vi "Write Page Button List Properties.vi"(8 "Error In":errorcluster, 10 "Button List Properties":T1[](array[typedef]), 11 "Custom Device Page .NET Ref In":refnum<k24>) -> (0 "Error Out":errorcluster, 3 "Custom Device Page .NET Ref Out":refnum<k24>)   [LabVIEW 2015, in "VeriStand Custom Device XML Parser.lvlib"]
doc: "Sets the properties for each button and sets the array of button properties to the page"
uses:
  VeriStand Custom Device XML Parser.lvlib
  NationalInstruments.VeriStand.XMLReader
  XML Controls/ButtonLists Properties.ctl
  XML Controls/Path Cluster.ctl
  XML Controls/Button Type.ctl
  XML Controls/Dependency Properties.ctl
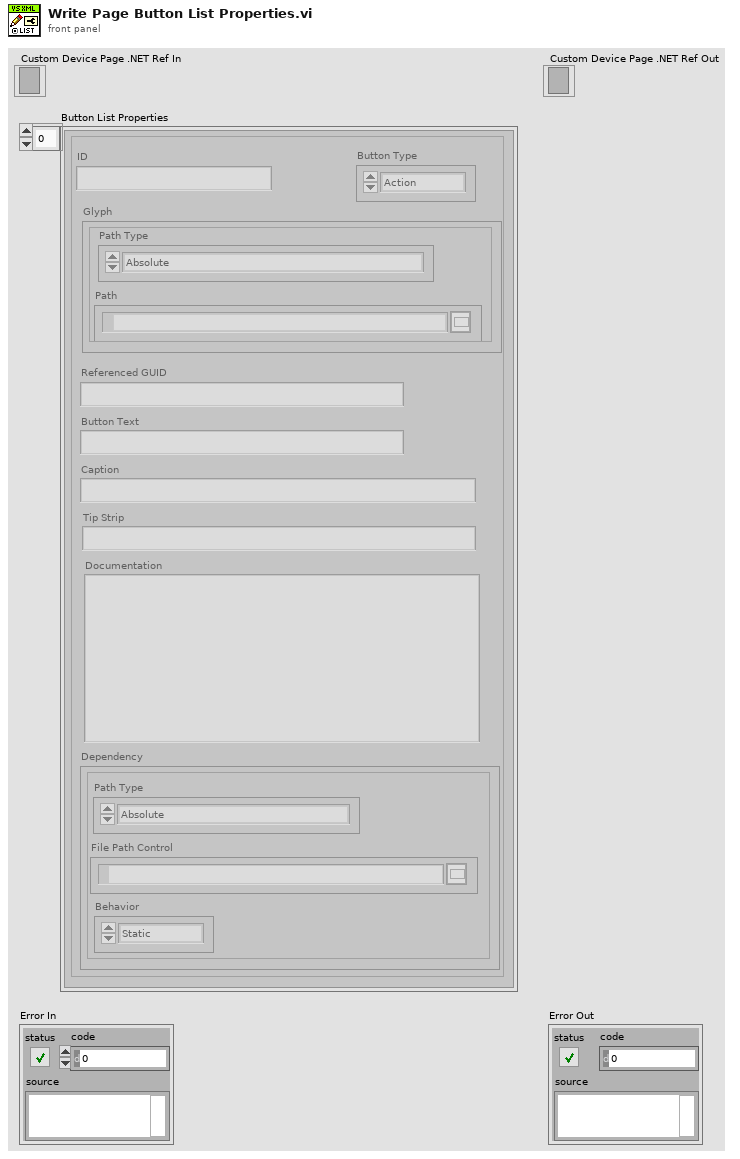
[diagram p1: front panel]
types:
  T1 = typedef "VeriStand Custom Device XML Parser.lvlib/ButtonLists Properties.ctl" = cluster{"ID":string, "Glyph":T2, "Button Type":T3, "Referenced GUID":string, "Button Text":string, "Caption":string, "Tip Strip":string, "Documentation":string, "Dependency":T4}
  T2 = typedef "VeriStand Custom Device XML Parser.lvlib/Path Cluster.ctl" = cluster{"Path":path, "Path Type":enum16{"Absolute", "To Base", "To Common Doc Dir", "To Application Data Dir"}}
  T3 = typedef "VeriStand Custom Device XML Parser.lvlib/Button Type.ctl" = enum16{"Action", "Dialog", "Page", "Notification", "Separator"}
  T4 = typedef "VeriStand Custom Device XML Parser.lvlib/Dependency Properties.ctl" = cluster{"File Path Control":path, "Path Type":enum16{"Absolute", "To Base", "To Common Doc Dir", "To Application Data Dir"}, "Behavior":enum16{"Static", "Dynamic"}}
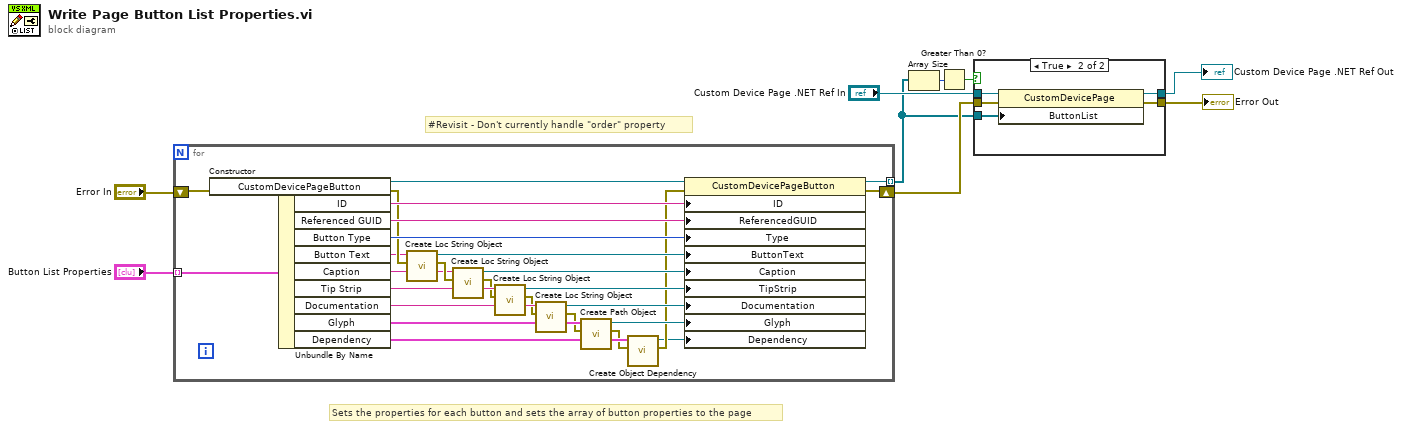
[diagram p0: block diagram]
diagram:
  # "Sets the properties for each button and sets the array of button properties to the page"
  # "#Revisit - Don't currently handle \"order\" property"
  n1 = for {
    tunnel: "Button List Properties" -> [w36] mode=indexing
    shift-right: [w15] -> w7
    shift-left: "Error In" -> [w35]
    tunnel: [w14] -> w1 mode=indexing
    n2 = constructor class="CustomDevicePageButton"(error in=w35) -> (reference out=w34:refnum<k24>, error out=w30:errorcluster)  [unwired: 2 in, 1 out]
    n3 = Unbundle By Name(w36) -> ("ID"=w33:string, "Referenced GUID"=w32:string, "Button Type"=w31:T3, "Button Text"=w29:string, "Caption"=w26:string, "Tip Strip"=w24:string, "Documentation"=w22:string, "Glyph"=w18:T2, "Dependency"=w13:T4)
    n4 = call "Create Loc String Object.vi"("Error In"=w30, "String Input"=w29) -> ("Error Out"=w27:errorcluster, "Loc String .NET Ref"=w28:refnum<k24>)  [unwired: 8 in]
    n5 = call "Create Loc String Object.vi"("Error In"=w27, "String Input"=w26) -> ("Error Out"=w23:errorcluster, "Loc String .NET Ref"=w25:refnum<k24>)  [unwired: 8 in]
    n6 = call "Create Loc String Object.vi"("Error In"=w23, "String Input"=w24) -> ("Error Out"=w21:errorcluster, "Loc String .NET Ref"=w20:refnum<k24>)  [unwired: 8 in]
    n7 = call "Create Loc String Object.vi"("Error In"=w21, "String Input"=w22) -> ("Error Out"=w17:errorcluster, "Loc String .NET Ref"=w19:refnum<k24>)  [unwired: 8 in]
    n8 = call "Create Path Object.vi"("Error In"=w17, "Path Data Cluster"=w18) -> ("Error Out"=w12:errorcluster, "Path .NET Ref"=w16:refnum<k24>)  [unwired: 8 in]
    n9 = call "Create Object Dependency.vi"("Error In"=w12, "Dependency Properties"=w13) -> ("Error Out"=w11:errorcluster, "Dependency .NET Ref Out"=w10:refnum<k24>)  [unwired: 8 in]
    n10 = property class="CustomDevicePageButton"(reference=w34, error in=w11, "ID"=w33, "ReferencedGUID"=w32, "Type"=w31, "ButtonText"=w28, "Caption"=w25, "TipStrip"=w20, "Documentation"=w19, "Glyph"=w16, "Dependency"=w10) -> (reference out=w14:refnum<k24>, error out=w15:errorcluster)
  }
  n11 = Array Size(array=w1) -> (size(s)=w3:i32)
  n12 = Greater Than 0?(x=w3) -> (x > 0?=w2:bool)
  n13 = case shown="True" w2 {
    tunnel: [w37 w43] -> w9
    tunnel: w1 -> [_ w42]
    tunnel: [w38 w41] -> w8
    tunnel: w7 -> [w37 w40]
    tunnel: "Custom Device Page .NET Ref In" -> [w38 w39]
    frame False {
    }
    frame True {
      n14 = property class="CustomDevicePage"(reference=w39, error in=w40, "ButtonList"=w42) -> (reference out=w41:refnum<k24>, error out=w43:errorcluster)
    }
  }
  "Error Out" <- w9
  "Custom Device Page .NET Ref Out" <- w8
